vi "GPSPathTracker.vi"() -> ()   [LabVIEW 2024]
uses:
  <vilib>/Instr/_visa.llb/VISA Configure Serial Port (Instr).vi
panel:
  out "PathHeading":dbl
  out "CTE":dbl
  out "NearPointIndex":i32
  in  "Y_Array":dbl[](array[numeric])
  in  "X_Array":dbl[](array[numeric])
  out "Altitude(m)":dbl
  out "Logitude(deg)":dbl
  out "Latitude(deg)":dbl
  in  "COM7":refnum<visa-resource-name>="COM3" caption="GPS_Com."
  out "True_Heading":dbl format="%#_15g"
  out "UTM X(E) INS":dbl format="%#_13g"
  out "UTM Y(N) INS":dbl format="%#_13g"
  out "GPS_Speed(kph)":dbl format="%#_g kph"
  in  "Stop":bool
  out "NMEA_Raw_Data":string
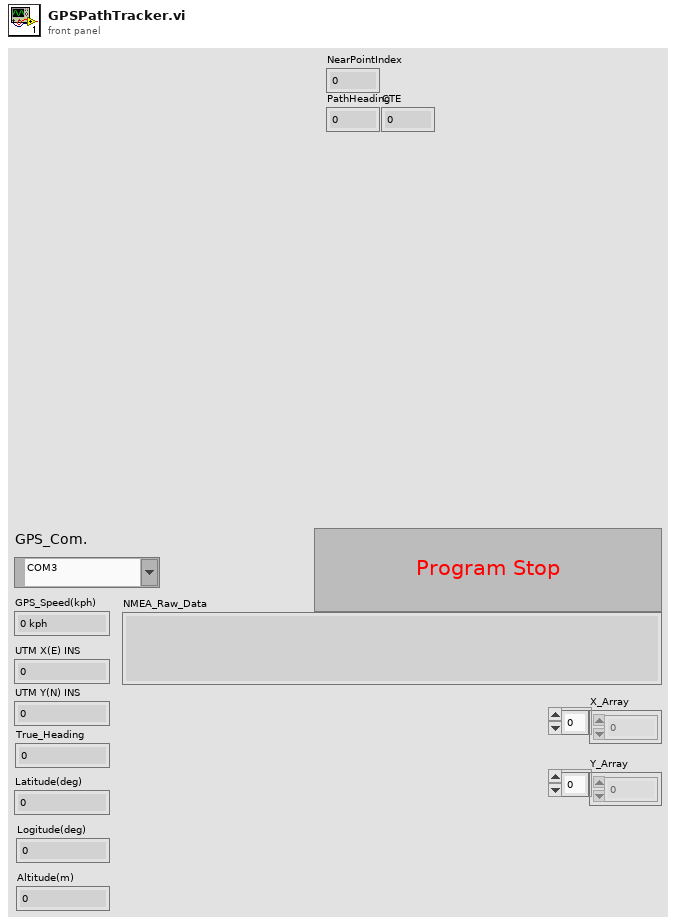
[diagram p1: front panel]
types:
  T1 = cluster{"oldest read timestamp":dbl, "latitude (deg)":dbl, "longitude (deg)":dbl, "ground speed (kph)":dbl, "true track angle (deg)":dbl, "altitude above mean sea level (m)":dbl}
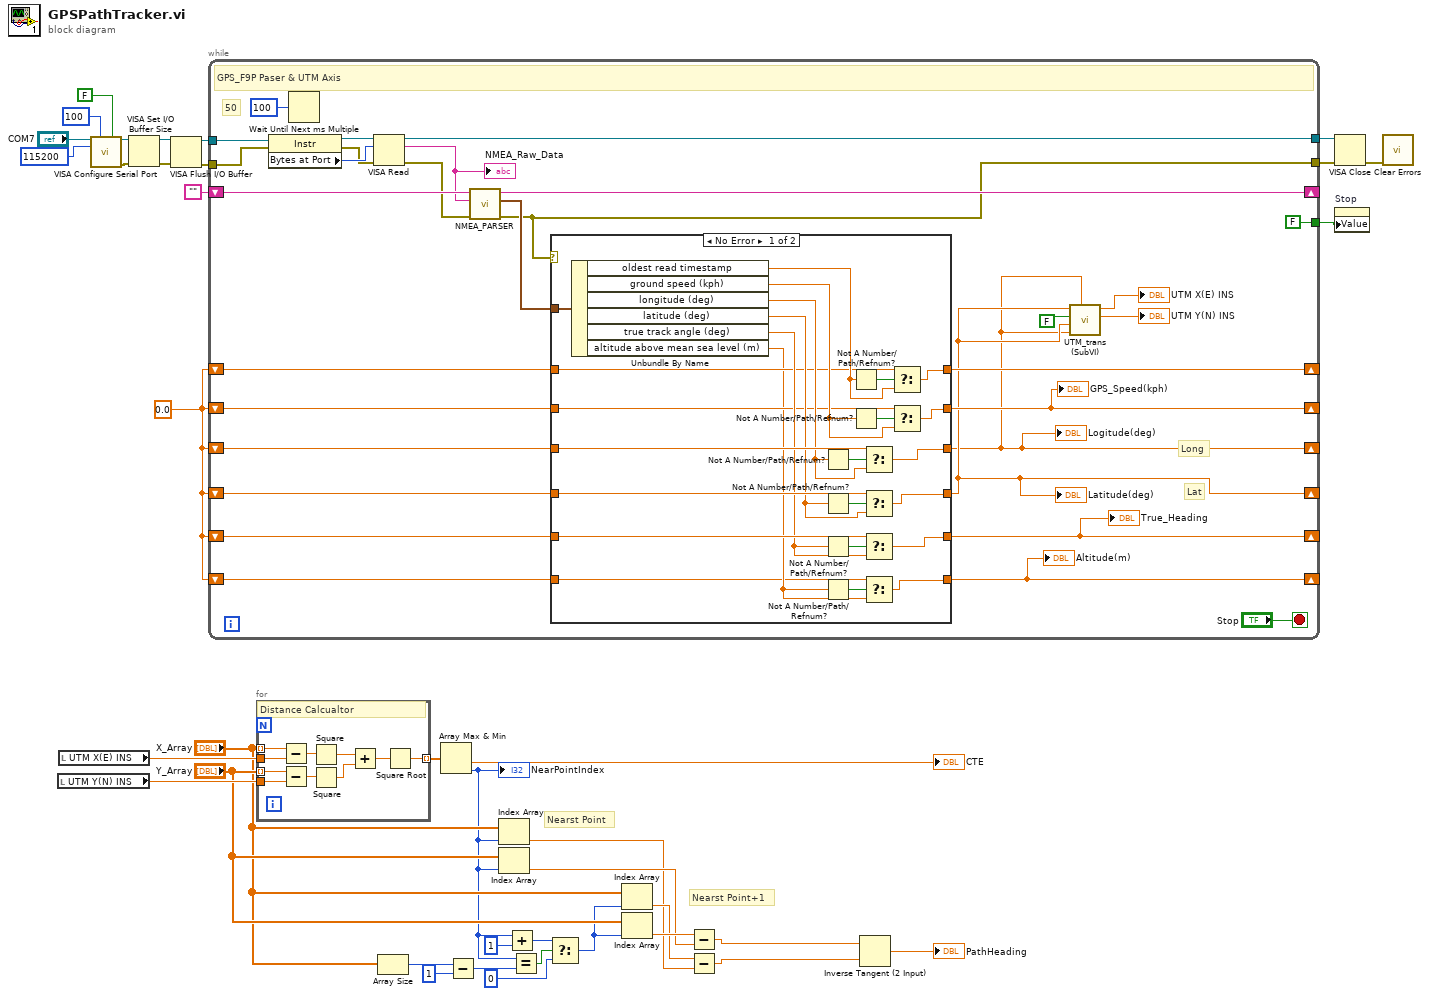
[diagram p0: block diagram]
diagram:
  w23 = 0.0 ("x")
  # "Nearst Point+1"
  # "Nearst Point"
  n1 = local read "UTM Y(N) INS"() -> (w21:dbl)
  n2 = local read "UTM X(E) INS"() -> (w22:dbl)
  n3 = call-poly "VISA Configure Serial Port"("VISA resource name"="COM7", "timeout (10sec)"=u32 100, "Enable Termination\nChar (T)"=FALSE ("Enable Termination\nChar (T)"), "baud rate (9600)"=u32 115200) -> ("VISA resource name out"=w29:refnum<visa-resource-name>, "error out"=w28:errorcluster)  [unwired: 10 in]
  n4 = VISA Set I/O Buffer Size(VISA resource name=w29, error in (no error)=w28) -> (VISA resource name out=w35:refnum<visa-resource-name>, error out=w34:errorcluster)  [unwired: 2 in]
  n5 = VISA Flush I/O Buffer(VISA resource name=w35, error in (no error)=w34) -> (VISA resource name out=w33:refnum<visa-resource-name>, error out=w32:errorcluster)  [unwired: 1 in]
  n6 = while {
    tunnel: w33 -> [w66]
    tunnel: w32 -> [w64]
    tunnel: [w68] -> w38
    tunnel: [w56] -> w36
    shift-right: [w57] -> _
    shift-left: "" -> [w61]
    shift-right: [w43] -> _
    shift-left: w23 -> [w55]
    shift-right: [w41] -> _
    shift-left: w23 -> [w54]
    shift-right: [w42] -> _
    shift-left: w23 -> [w53]
    shift-right: [w49] -> _
    shift-left: w23 -> [w52]
    shift-right: [w48] -> _
    shift-left: w23 -> [w51]
    tunnel: [FALSE] -> w30
    shift-right: [w39] -> _
    shift-left: w23 -> [w40]
    stop <- "Stop" stop-if-true
    # "Lat"
    # "Long"
    # "50"
    # "GPS_F9P Paser & UTM Axis"
    n7 = property class="Instr"(reference=w66, error in=w64) -> (reference out=w65:refnum<visa-resource-name>, error out=w63:errorcluster, "Bytes at Port"=w67:u32)
    n8 = Wait Until Next ms Multiple(millisecond multiple=u32 100) -> ()  [unwired: 1 out]
    n9 = VISA Read(VISA resource name=w65, byte count=w67, error in (no error)=w63) -> (VISA resource name out=w68:refnum<visa-resource-name>, read buffer=w60:string, error out=w58:errorcluster)  [unwired: 1 out]
    "NMEA_Raw_Data" <- w60
    n10 = call "NMEA_PARSER.vi"("previous partial sentence"=w61, "sensor data"=w60, "error in (no error)"=w58) -> ("remaining partial sentence"=w57:string, "GPS data"=w59:T1, "error out"=w56:errorcluster)  [unwired: 5 in]
    n11 = case shown="No Error" w56 {
      tunnel: w59 -> [w93 _]
      tunnel: w54 -> [w89 w99]
      tunnel: w53 -> [w88 w98]
      tunnel: w52 -> [w87 w97]
      tunnel: [w83 w99] -> w41
      tunnel: [w82 w98] -> w42
      tunnel: [w81 w97] -> w49
      tunnel: w55 -> [w78 w96]
      tunnel: [w77 w96] -> w43
      tunnel: w51 -> [w74 w95]
      tunnel: [w73 w95] -> w48
      tunnel: [w70 w94] -> w39
      tunnel: w40 -> [w69 w94]
      frame No Error {
        n12 = Unbundle By Name(w93) -> ("oldest read timestamp"=w75:dbl, "ground speed (kph)"=w79:dbl, "longitude (deg)"=w86:dbl, "latitude (deg)"=w85:dbl, "true track angle (deg)"=w84:dbl, "altitude above mean sea level (m)"=w71:dbl)
        n13 = Not A Number/Path/Refnum?(number/path/refnum=w86) -> (NaN/Path/Refnum?=w92:bool)
        n14 = Not A Number/Path/Refnum?(number/path/refnum=w85) -> (NaN/Path/Refnum?=w91:bool)
        n15 = Not A Number/Path/Refnum?(number/path/refnum=w84) -> (NaN/Path/Refnum?=w90:bool)
        n16 = Not A Number/Path/Refnum?(number/path/refnum=w71) -> (NaN/Path/Refnum?=w72:bool)
        n17 = Not A Number/Path/Refnum?(number/path/refnum=w75) -> (NaN/Path/Refnum?=w76:bool)
        n18 = Not A Number/Path/Refnum?(number/path/refnum=w79) -> (NaN/Path/Refnum?=w80:bool)
        n19 = Select(t=w89, s=w92, f=w86) -> (s? t:f=w83:dbl)
        n20 = Select(t=w88, s=w91, f=w85) -> (s? t:f=w82:dbl)
        n21 = Select(t=w87, s=w90, f=w84) -> (s? t:f=w81:dbl)
        n22 = Select(t=w69, s=w72, f=w71) -> (s? t:f=w70:dbl)
        n23 = Select(t=w74, s=w76, f=w75) -> (s? t:f=w73:dbl)
        n24 = Select(t=w78, s=w80, f=w79) -> (s? t:f=w77:dbl)
      }
      frame Error {
        # "Invalid data points."
      }
    }
    "True_Heading" <- w49
    "GPS_Speed(kph)" <- w43
    "Latitude(deg)" <- w42
    "Logitude(deg)" <- w41
    "Altitude(m)" <- w39
    n25 = call "UTM_trans (SubVI).vi"("Long_Deg"=w41, "long"=w41, "lat"=w42, "East?West?"=FALSE, "Lat_Deg"=w42) -> ("UTM_Y(Northing)"=→"UTM Y(N) INS":dbl, "UTM_X(Easting)"=→"UTM X(E) INS":dbl)  [unwired: 2 out]
  }
  n26 = for {
    tunnel: "X_Array" -> [w109] mode=indexing
    tunnel: "Y_Array" -> [w108] mode=indexing
    tunnel: w22 -> [w107]
    tunnel: w21 -> [w106]
    tunnel: [w100] -> w20 mode=indexing
    # "Distance Calcualtor"
    n27 = Subtract(x=w109, y=w107) -> (x-y=w105:dbl)
    n28 = Subtract(x=w108, y=w106) -> (x-y=w104:dbl)
    n29 = Square(x=w105) -> (x^2=w103:dbl)
    n30 = Square(x=w104) -> (x^2=w102:dbl)
    n31 = Add(x=w103, y=w102) -> (x+y=w101:dbl)
    n32 = Square Root(x=w101) -> (sqrt(x)=w100:dbl)
  }
  n33 = Array Size(array="X_Array") -> (size(s)=w10:i32)
  n34 = Array Max & Min(array=w20) -> (min value=→"CTE":dbl, min index (indices)=w11:i32)  [unwired: 2 out]
  "NearPointIndex" <- w11
  n35 = Subtract(x=w10, y=1) -> (x-y=w9:i32)
  n36 = Index Array(array="X_Array", index=w11) -> (element=w4:dbl)
  n37 = Index Array(array="Y_Array", index=w11) -> (element=w6:dbl)
  n38 = Add(x=w11, y=1) -> (x+y=w16:i32)
  n39 = Equal?(x=w11, y=w9) -> (x = y?=w12:bool)
  n40 = Select(t=w16, s=w12, f=0) -> (s? t:f=w15:i32)
  n41 = Index Array(array="X_Array", index=w15) -> (element=w5:dbl)
  n42 = Index Array(array="Y_Array", index=w15) -> (element=w7:dbl)
  n43 = Subtract(x=w7, y=w6) -> (x-y=w3:dbl)
  n44 = Subtract(x=w5, y=w4) -> (x-y=w2:dbl)
  n45 = Inverse Tangent (2 Input)(1:w2, 2:w3) -> (0:→"PathHeading":dbl)
  n46 = VISA Close(VISA resource name=w38, error in (no error)=w36) -> (error out=w37:errorcluster)
  n47 = property on="Stop" class="Bool (strict)"("Value"=w30) -> ()  [unwired: 2 in, 2 out]
  n48 = call <vilib>:"Clear Errors.vi"("error in (no error)"=w37) -> ()  [unwired: 5 in, 2 out]
